vi "Omni Fieldcentric.vi"(7 "Point Robot":bool, 8 "reinit?":bool, 9 "axis 1 (x)":dbl, 10 "axis 2 (y)":dbl, 11 "Steer Target Angle":dbl) -> (1 "Translation X":dbl, 2 "Translation Y":dbl, 3 "Rotation":dbl)   [LabVIEW 2013]
uses:
  Common Code/Change Detect Boolean.vi
  Robot Global Data.vi
  <vilib>/Rock Robotics/WPI/Gyro/WPI_GyroRefNum Registry Get.vi
  <vilib>/Rock Robotics/WPI/Gyro/WPI_GyroGetAngle.vi
panel:
  in  "steer axis 2":dbl
  out "Rotation 2":dbl
  out "Steer Target Angle 2":dbl
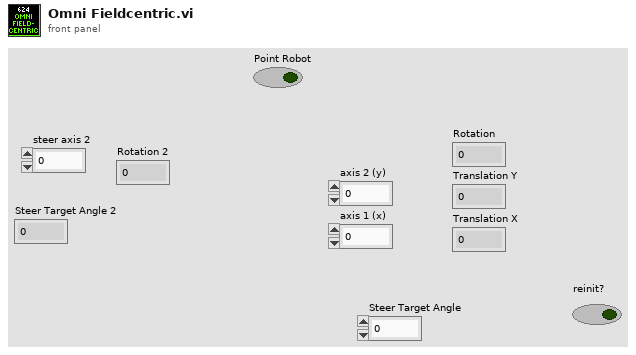
[diagram p1: front panel]
types:
  T1 = typedef "Dashboard UDP Packet.ctl" = cluster{"Camera":T2, "Gyro":T3, "Encoder":T5, "Auto Shift":T6, "Auton":T7, "Drive/Ramp X":dbl, "Drive/Ramp Y":dbl, "Drive/Battery Cutoff":dbl, "Pressure/Compressor Min Voltage":dbl, "Pressure/Compressor Delay":dbl, "Controller/Strafe Correction":bool, "Shooter":T8, "Rollers":T9, "Abort":bool, "Finish":bool, "IR Halo Sustain Time":dbl, "Disable Compressor":bool, "Center Omni Drive Delay":i32, "Vision Mode":T10, "Radius Throttle":bool, "Fieldcentric":T11, "Roll":T12, "Stick Deadband":dbl}
  T2 = typedef "Camera Controls.ctl" = cluster{"Camera/View Angle X":dbl, "Camera/Goal Track Timeout":dbl, "Camera/View Angle Y":dbl, "Camera/Goal Exposure":dbl, "Camera/Vision Receive Timeout":dbl, "Camera/Offset 1":dbl, "Camera/Offset 2":dbl}
  T3 = typedef "Gyro Controls.ctl" = cluster{"Gyro/Angle Tolerance":dbl, "Gyro/Steer Closeness Threshold":dbl, "Steer PID":T4, "Steer Close PID":T4}
  T4 = typedef "PID Params.ctl" = cluster{"max":dbl, "min":dbl, "P":dbl, "I":dbl, "D":dbl}
  T5 = typedef "Encoder Controls.ctl" = cluster{"Encoders/Reset":bool, "Encoders/Omni Constant":dbl, "Encoders/Omni Tick Constant":dbl, "Encoders/Left Constant":dbl, "Encoders/Right Constant":dbl, "Encoders/Right Tick Constant":dbl}
  T6 = typedef "Auto Shift Controls.ctl" = cluster{"AutoShift/Upshift Throttle Accel":dbl, "AutoShift/Speed Threshold":dbl, "AutoShift/Upshift Throttle":dbl, "AutoShift/Upshift Accel":dbl, "AutoShift/Downshift Accel":dbl, "AutoShift/Downshift Throttle":dbl, "AutoShift/Delay":dbl, "AutoShift/Enabled":bool}
  T7 = typedef "Auton Controls.ctl" = cluster{"Auton/Left Shoot X-Coord":dbl, "Auton/Right Shoot X-Coord":dbl, "DistDrive/Distance Stop Threshold":dbl, "DistDrive/Max Stop Speed":dbl, "Auton/Back Piston Time":dbl, "Auton/Manual Hot":bool, "Auton/Manual Hot Right":bool, "Default X PID":T4, "Default Y PID":T4}
  T8 = typedef "Shooter Controls.ctl" = cluster{"Shooter/Reset Time":dbl, "Shooter/Release Delay":dbl, "Shooter/Pressure Steady Time":dbl, "Shooter/Misfire Delay":dbl, "Shooter/Ball Settle Time":dbl, "Shooter/Line IR Delay":dbl, "Pressure/Upper PSI Time":dbl, "Pressure/Lower PSI Time":dbl, "Shooter/Punch Delay":dbl, "Shooter/Target Pressure":dbl, "Pressure/Line B":dbl, "Pressure/Line M":dbl, "Pressure/Shooter M":dbl, "Pressure/Shooter B":dbl, "Halo Time":dbl, "Soft Release Delay":dbl, "Soft Unpin Delay":dbl, "Soft Shoot Delay":dbl}
  T9 = typedef "Roller Controls.ctl" = cluster{"Roller/Load IRs Verify Time":dbl, "Roller/Center IR Latch Time":dbl, "Roller/Speed Front":dbl, "Roller/Speed Back":dbl, "Roller/Entry Timeout":dbl, "Roller/To Center Timeout":dbl, "Roller/Sustain Time":dbl, "Roller/Verify Center Time":dbl}
  T10 = typedef "Vision Mode.ctl" = enum16{"Normal", "Extreme Left", "Extreme Right"}
  T11 = typedef "Fieldcentric Controls.ctl" = cluster{"Relative Angle":bool, "Point Robot":bool, "X/Y ratio low":dbl, "Steering Gain":dbl, "Force Omni Down":bool, "Enable":bool, "X/Y ratio high":dbl}
  T12 = typedef "Roll Maneuver.ctl" = cluster{"X 1":dbl, "Y 1":dbl, "Y 2":dbl, "X 2":dbl, "Y 3":dbl, "X 3":dbl, "Time 1":i32, "Time 2":i32, "Time 3":i32, "Angle Start":dbl, "Angle End":dbl, "Angle Linearity":dbl}
  T13 = typedef "Drivetrain Status.ctl" = cluster{"Mode":T14, "X":dbl, "Y":dbl, "Steer":dbl, "Low Gear":bool, "Omni":bool}
  T14 = typedef "DT Mode.ctl" = enum16{"Manual", "Gyro Steer", "Distance Drive", "Fieldcentric", "Roll Maneuver", "Alt Roll Maneuver"}
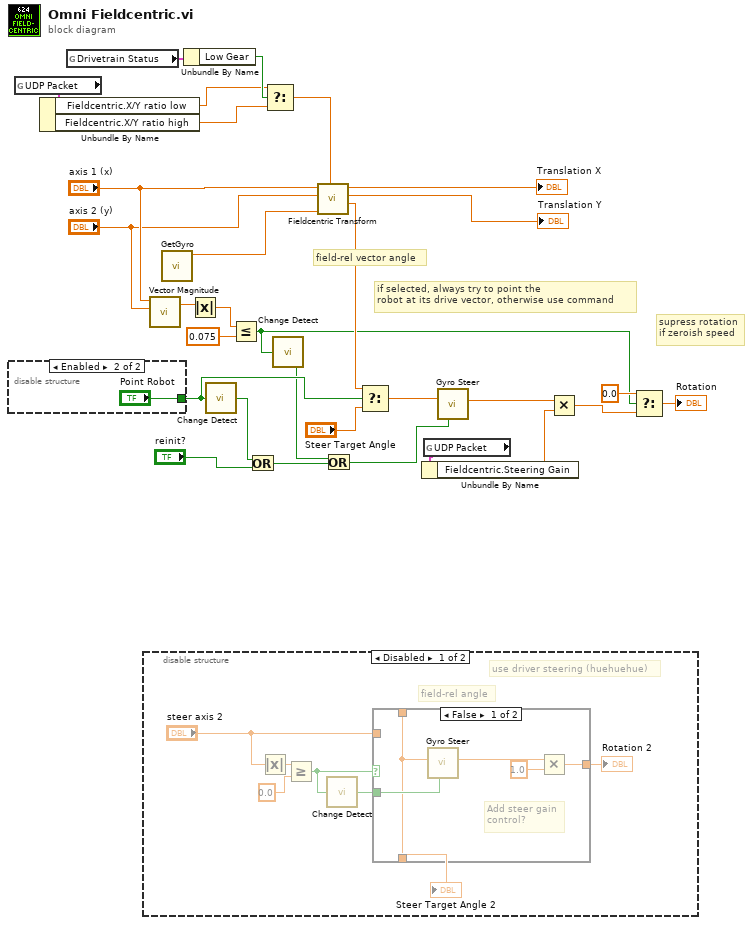
[diagram p0: block diagram]
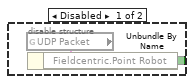
[diagram p2: hidden frame]
diagram:
  # "supress rotation\nif zeroish speed"
  # "if selected, always try to point the \nrobot at its drive vector, otherwise use command"
  # "field-rel vector angle"
  n1 = disable-structure shown="Enabled" {
    disable-tunnel: [w31 "Point Robot"] -> w20
    frame Disabled {
      n2 = global read "Robot Global Data.vi" "UDP Packet"() -> (w32:T1)
      n3 = Unbundle By Name(w32) -> ("Fieldcentric.Point Robot"=w31:bool)
    }
    frame Enabled {
    }
  }
  n4 = global read "Robot Global Data.vi" "UDP Packet"() -> (w27:T1)
  n5 = Unbundle By Name(w27) -> ("Fieldcentric.X/Y ratio low"=w17:dbl, "Fieldcentric.X/Y ratio high"=w16:dbl)
  n6 = global read "Robot Global Data.vi" "Drivetrain Status"() -> (w19:T13)
  n7 = disable-structure shown="Disabled" {
    frame Disabled {
      # "use driver steering (huehuehue)"
      # "field-rel angle"
      n8 = Absolute Value(x="steer axis 2") -> (abs(x)=w34:dbl)
      n9 = Greater Or Equal?(x=w34, y=0.0) -> (x >= y?=w38:bool)
      n10 = call-poly "Change Detect.vi"("In"=w38) -> ("Changed?"=w39:bool)
      n11 = case shown="False" w38 {
        tunnel: [w42 w46] -> w36
        tunnel: "steer axis 2" -> [_ w46]
        tunnel: w39 -> [w45 _]
        tunnel: _ -> [w44 _]
        tunnel: [w44 _] -> w40
        frame False {
          # "Add steer gain\ncontrol?"
          n12 = call "Gyro Steer.vi"("reinitialize? (F)"=w45, "Target Angle"=w44) -> ("Steering Out"=w43:dbl)  [unwired: 8 in, 1 out]
          n13 = Multiply(x=w43, y=1.0) -> (x*y=w42:dbl)
        }
        frame True {
        }
      }
      "Rotation 2" <- w36
      "Steer Target Angle 2" <- w40
    }
    frame Enabled {
    }
  }
  n14 = call "Vector Magnitude.vi"("Y"="axis 2 (y)", "X"="axis 1 (x)") -> ("Magnitude"=w12:dbl)  [unwired: 3 in]
  n15 = call "GetGyro.vi"() -> ("Angle"=w28:dbl)  [unwired: 9 in, 2 out]
  n16 = Unbundle By Name(w19) -> ("Low Gear"=w18:bool)
  n17 = Absolute Value(x=w12) -> (abs(x)=w11:dbl)
  n18 = call-poly "Change Detect.vi"("In"=w20) -> ("Changed?"=w3:bool)
  n19 = Less Or Equal?(x=w11, y=0.075) -> (x <= y?=w7:bool)
  n20 = Or(x=w3, y="reinit?") -> (x .or. y?=w6:bool)
  n21 = Select(t=w17, s=w18, f=w16) -> (s? t:f=w1:dbl)
  n22 = call-poly "Change Detect.vi"("In"=w7) -> ("Changed?"=w5:bool)
  n23 = call "Fieldcentric Transform.vi"("X/Y Ratio"=w1, "Gyro Angle"=w28, "Y"="axis 2 (y)", "X"="axis 1 (x)") -> ("Field-rel angle"=w23:dbl, "Vector Y"=→"Translation Y":dbl, "X Out"=→"Translation X":dbl)  [unwired: 4 in, 1 out]
  n24 = Or(x=w5, y=w6) -> (x .or. y?=w4:bool)
  n25 = Select(t=w23, s=w20, f="Steer Target Angle") -> (s? t:f=w22:dbl)
  n26 = global read "Robot Global Data.vi" "UDP Packet"() -> (w25:T1)
  n27 = Unbundle By Name(w25) -> ("Fieldcentric.Steering Gain"=w24:dbl)
  n28 = call "Gyro Steer.vi"("reinitialize? (F)"=w4, "Target Angle"=w22) -> ("Steering Out"=w26:dbl)  [unwired: 8 in, 1 out]
  n29 = Multiply(x=w26, y=w24) -> (x*y=w10:dbl)
  n30 = Select(t=0.0, s=w7, f=w10) -> (s? t:f=→"Rotation":dbl)
